vi "RemoveBorder.vi"(1 "Larger Image":u8[][](array[numeric]), 2 "Original Image":u8[][](array[numeric])) -> (0 "Subset":u8[][](array[numeric]))   [LabVIEW 2024]
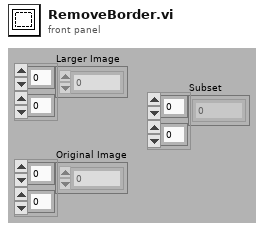
[diagram p1: front panel]
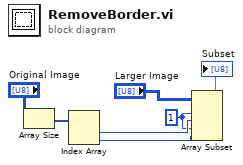
[diagram p0: block diagram]
diagram:
  w1 = 1 ("index")
  n1 = Array Size(array="Original Image") -> (size(s)=w2:i32[])
  n2 = Index Array(array=w2) -> (element #1=w3:i32, element #2=w4:i32)  [unwired: 2 in]
  n3 = Array Subset(array="Larger Image", index (row)=w1, length (row)=w3, index (col)=w1, length (col)=w4) -> (→"Subset":u8[][])
